vi "Example Threshold.vi"() -> ()   [LabVIEW 2010]
uses:
  C:/tf/play/labview/Tinkerforge.dll
panel:
  in  "stop":bool
  out "callback counter":i32
  out "last current (A)":sgl
  in  "uid":string="amb"
  in  "port":i32=4223
  in  "host":string="localhost"
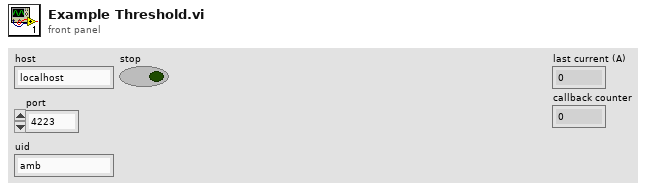
[diagram p1: front panel]
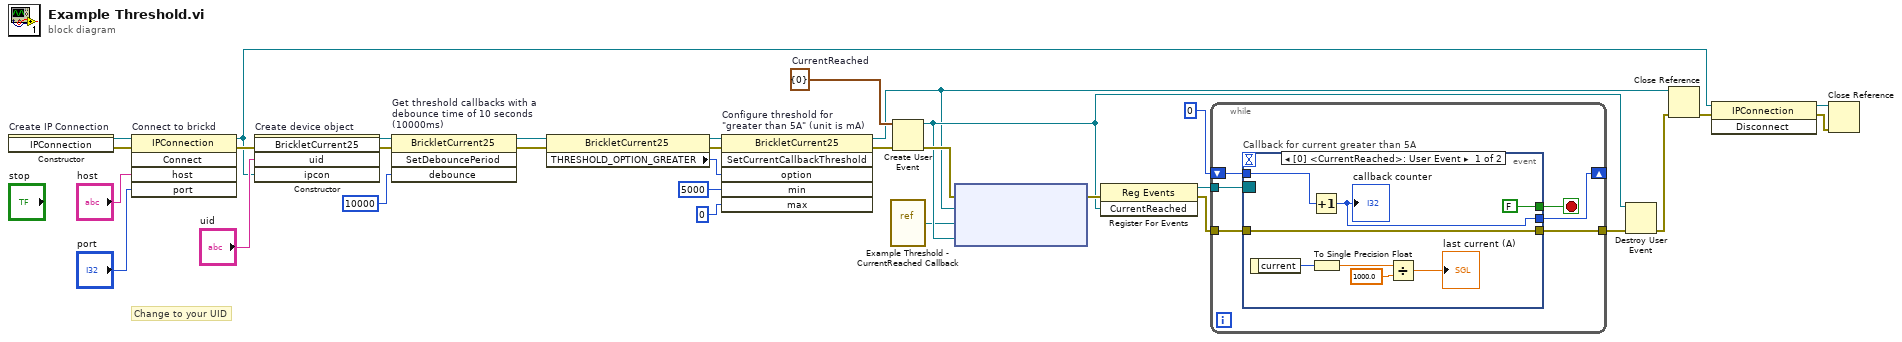
[diagram p0: block diagram]
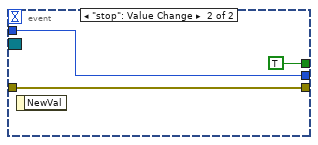
[diagram p2: hidden frame]
diagram:
  w16 = cluster{"current":i16} {"current"=0}  # CurrentReached
  # "Change to your UID"
  n1 = constructor on="Create IP Connection" class="IPConnection"() -> (reference out=w32:refnum<k24>, error out=w2:errorcluster)  [unwired: 3 in, 1 out]
  n2 = invoke on="Connect to brickd" class="IPConnection" method="Connect"(reference=w32, error in=w2, "host"="host", "port"="port") -> (reference out=w25:refnum<k24>, error out=w28:errorcluster)  [unwired: 1 in, 3 out]
  n3 = constructor on="Create device object" class="BrickletCurrent25"(error in=w28, "uid"="uid", "ipcon"=w25) -> (reference out=w14:refnum<k24>, error out=w15:errorcluster)  [unwired: 2 in, 3 out]
  n4 = invoke on="Get threshold callbacks with a\ndebounce time of 10 seconds\n(10000ms)" class="BrickletCurrent25" method="SetDebouncePeriod"(reference=w14, error in=w15, "debounce"=i64 10000 ("period")) -> (reference out=w6:refnum<k24>, error out=w8:errorcluster)  [unwired: 1 in, 2 out]
  n5 = property class="BrickletCurrent25"(reference=w6, error in=w8) -> (reference out=w5:refnum<k24>, error out=w7:errorcluster, "THRESHOLD_OPTION_GREATER"=w4:u16)
  n6 = invoke on="Configure threshold for\n\"greater than 5A\" (unit is mA)" class="BrickletCurrent25" method="SetCurrentCallbackThreshold"(reference=w5, error in=w7, "option"=w4, "min"=i16 5000, "max"=i16 0) -> (reference out=w12:refnum<k24>, error out=w11:errorcluster)  [unwired: 1 in, 4 out]
  n7 = vi-ref "Example Threshold - CurrentReached Callback.vi"() -> ("vi reference"=w1:refnum<vi>)
  n8 = Create User Event(user event datatype=w16, error in=w11) -> (user event=w18:refnum<user-event>, error out=w23:errorcluster)
  n9 = node ("Register Event Callback")(w23, w12, w1, w18) -> (w22:errorcluster)  [unwired: 1 in, 1 out]
  n10 = register-events(error in=w22, w18) -> (reference out=w21:refnum<event-registration>, error out=w19:errorcluster)  [unwired: 1 in]
  n11 = while {
    tunnel: w21 -> [w38]
    tunnel: [w37] -> w20
    tunnel: w19 -> [w36]
    shift-right: [w34] -> _
    shift-left: 0 -> [w35]
    stop <- w33 stop-if-true
    n12 = event "Callback for current greater than 5A" shown="[0] <CurrentReached>: User Event" {
      selector: w38 -> [_ _]
      dyn-events: _ -> [_ _]
      timeout: _ -> [_ _]
      tunnel: [w43 w48] -> w37
      tunnel: w36 -> [w43 w48]
      tunnel: w35 -> [w41 w47]
      tunnel: [w40 w47] -> w34
      tunnel: [FALSE TRUE] -> w33
      event User Event {
        n13 = event-data() -> ("current"=w44:i16)  [unwired: 1 in]
        n14 = Increment(x=w41) -> (x+1=w40:i32)
        "callback counter" <- w40
        n15 = To Single Precision Float(number=w44) -> (single precision float=w45:sgl)
        n16 = Divide(x=w45, y=sgl 1000.0) -> (x/y=→"last current (A)":sgl)
      }
      event "stop": Value Change {
        n17 = event-data() -> ()  [unwired: 1 in, 1 out]
      }
    }
  }
  n18 = Destroy User Event(user event=w18, error in=w20) -> (error out=w17:errorcluster)
  n19 = Close Reference(reference=w12, error in (no error)=w17) -> (error out=w27:errorcluster)
  n20 = invoke class="IPConnection" method="Disconnect"(reference=w25, error in=w27) -> (reference out=w24:refnum<k24>, error out=w26:errorcluster)  [unwired: 1 in, 1 out]
  n21 = Close Reference(reference=w24, error in (no error)=w26) -> ()  [unwired: 1 out]
